vi "Check_Execution_Row.vi"(0 "Execution Row":T1 {"Row Duration (mins)" format="%#.1f"; "Row No" min=0; "Trace Gas Concentration (%)" min=0.0 format="%#.2f"; "Emission Rate (l/min)" format="%#.2f"; "Tunnel Speed" format="%#.2f"; "Start X" format="%#.2f"; "Start Y" format="%#.2f"; "Start Z" format="%#.2f"; "End X" format="%#.2f"; "End Y" format="%#.2f"; "End Z" format="%#.2f"; "Averaging time (min)" min=0.0 format="%#.2f"}, 3 "Synchronization Start No":i32=1 min=1 max=100, 4 "Row Index":i32, 5 "Max Tunnel Speed":dbl format="%.2f") -> (6 "Editted Row":bool, 7 "Execution Row Out":T1 {"Row Duration (mins)" format="%#.1f"; "Row No" min=0; "Trace Gas Concentration (%)" min=0.0 format="%#.2f"; "Emission Rate (l/min)" format="%#.2f"; "Tunnel Speed" format="%#.2f"; "Start X" format="%#.2f"; "Start Y" format="%#.2f"; "Start Z" format="%#.2f"; "End X" format="%#.2f"; "End Y" format="%#.2f"; "End Z" format="%#.2f"; "Averaging time (min)" min=0.0 format="%#.2f"}, 9 "Continue?":bool, 10 "Error Comments":string)   [LabVIEW 2014]
uses:
  Traverse_cluster.ctl
  Spacing.ctl
  Controls/Multi_run_mode.ctl
  Controls/User_Specific_mode.ctl
  Controls/Home.ctl
  Controls/Tunnel_Coordinates.ctl
  ADAM Client/Sub VIs/ADAM Controls/Channel_names.ctl
  Globals/Extra_Commands_Global.vi
  Globals/Constants_global.vi
  Globals/Trav_pos_global.vi
panel:
  out "Traverse line Out":T1 {"Row Duration (mins)" format="%#.1f"; "Row No" min=0; "Trace Gas Concentration (%)" min=0.0 format="%#.2f"; "Emission Rate (l/min)" format="%#.2f"; "Tunnel Speed" format="%#.2f"; "Start X" format="%#.2f"; "Start Y" format="%#.2f"; "Start Z" format="%#.2f"; "End X" format="%#.2f"; "End Y" format="%#.2f"; "End Z" format="%#.2f"; "Averaging time (min)" min=0.0 format="%#.2f"}
  out "Fixed Axis":bool[](array[boolean])
  out "Filenames":string[](array[string])
  out "Current Sync Number":i32
  out "Checks":string[](array[string])
  in  "Edit in Excel":bool
  in  "OK":bool
  # "X           Y            Z"
  # "Start"
  # "End"
  # "X           Y            Z"
  # "Start"
  # "End"
  # "X           Y            Z"
  # "Start"
  # "End"
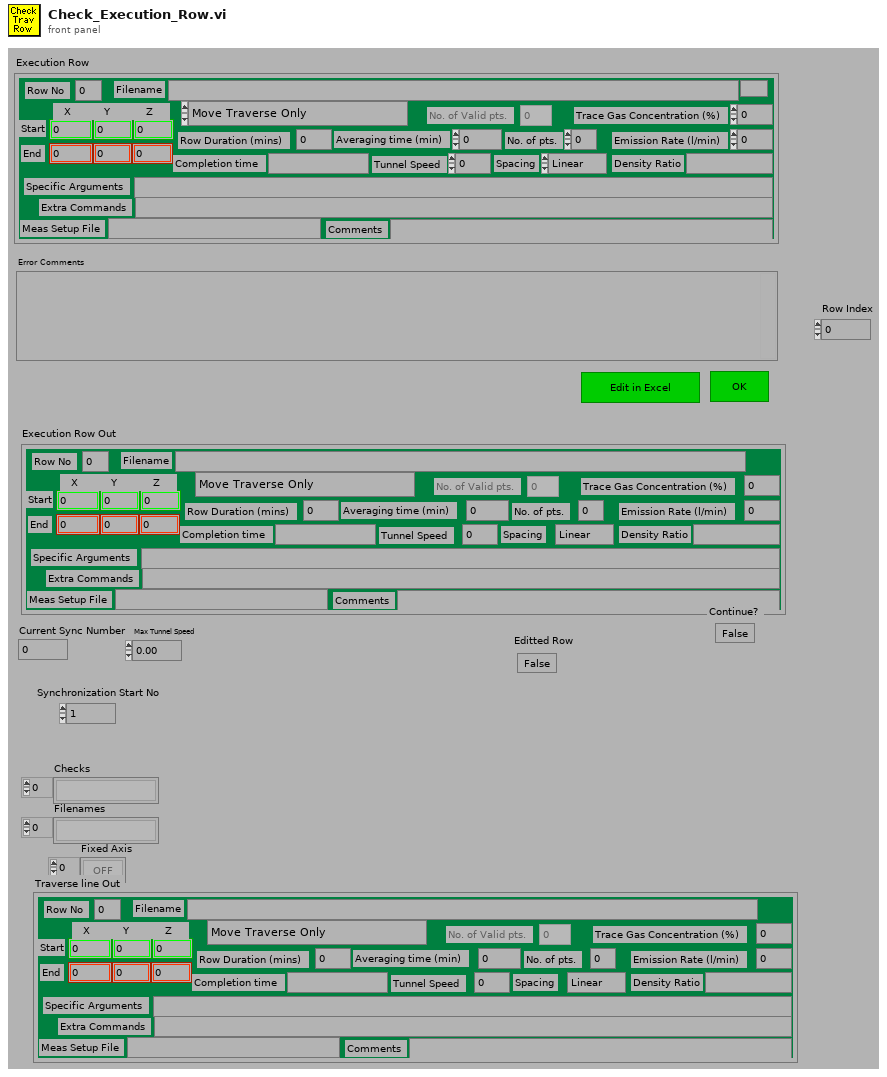
[diagram p1: front panel]
types:
  T1 = typedef "Traverse_cluster.ctl" = cluster{"Start X":dbl, "Start Y":dbl, "Start Z":dbl, "End X":dbl, "End Y":dbl, "End Z":dbl, "No. of pts.":i32, "Spacing":T2, "Filename":path, "Tunnel Speed":dbl, "Averaging time (min)":dbl, "Extra Commands":string, "Specific Arguments":string, "Emission Rate (l/min)":dbl, "Trace Gas Concentration (%)":dbl, "Density Ratio":string, "Comments":string, "Row No":i32, "Row Type Selector":T3, "Completion time":string, "Row Duration (mins)":dbl, "No. of Valid pts.":i32, "Meas Setup File":string}
  T2 = typedef "Spacing.ctl" = enum16{"Linear", "Log", "Gauss", "Specified", "N/A"}
  T3 = typedef "Multi_run_mode.ctl" = enum16{"Move Traverse Only", "Set Tunnel Speed Only", "Set Source Only", "Set Measurement Conditions", "Single Measurement", "Vertical Profile", "Lateral Profile", "Longitudinal Profile", "Explore Volume", "Multi-Axis Profile", "Auto Calibrate", "Meas Fast FID Bkgnd", "Check Beam Power", "Scanning Valve Measurement", "Run VI Named:", "Set ADAM Ch", "Wait (minutes)", "Send Message", "Synchronize With:", "Fall Back to this Row", "Turn Off Row Repeating", "Blank Row", "Traverse 3D Volume"}
  T4 = enum16{"All Channel Names", "Valid Channel Names"}
  T5 = typedef "User_Specific_mode.ctl" = enum16{"Check VI only", "Run VI"}
  T6 = typedef "Home.ctl" = enum16{"Don't Home", "Home  +X", "Home  -X", "Home  +Y", "Home  -Y", "Home  +Z", "Home  -Z"}
  T7 = typedef "Tunnel_Coordinates.ctl" = enum16{"Work in Tunnel Coordinates", "Work in Model Coordinates"}
  T8 = enum16{"Zero or one", "One", "Zero or more", "One or more"}
  T9 = typedef "Channel_names.ctl" = enum16{"Active Only", "Active + Off", "All Channels"}
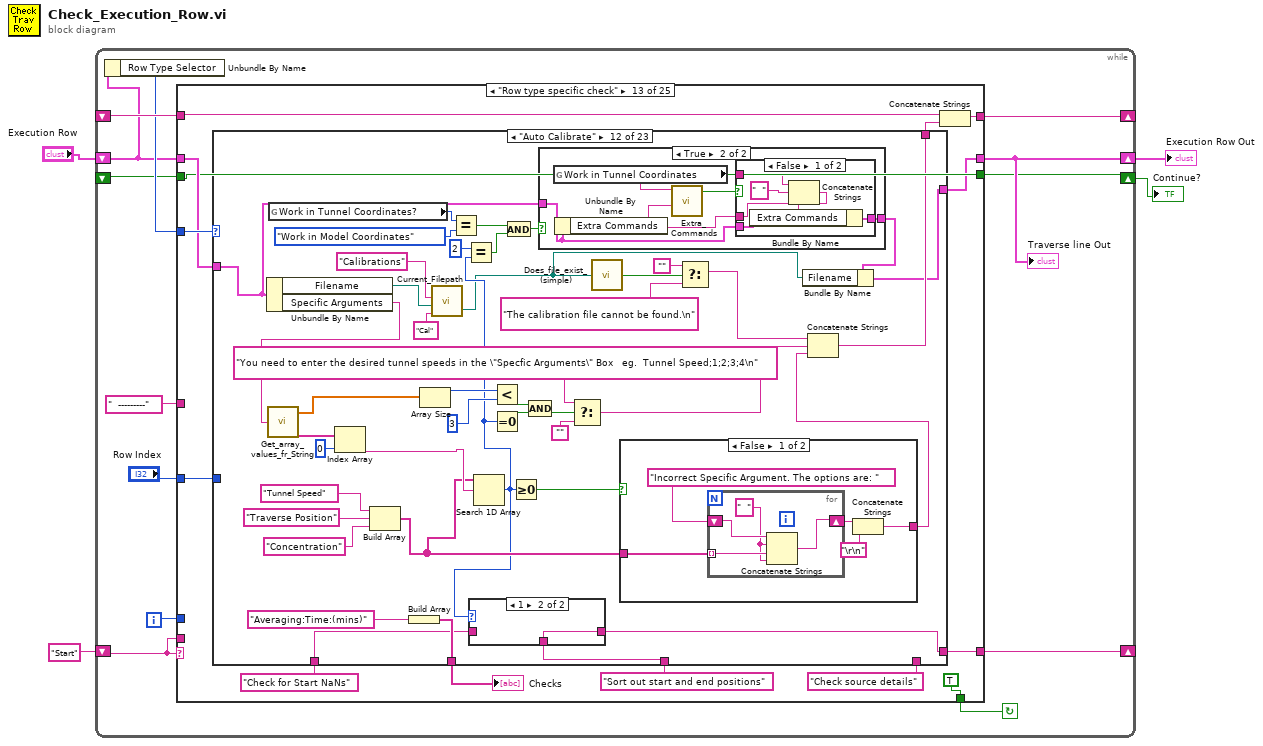
[diagram p0: block diagram]
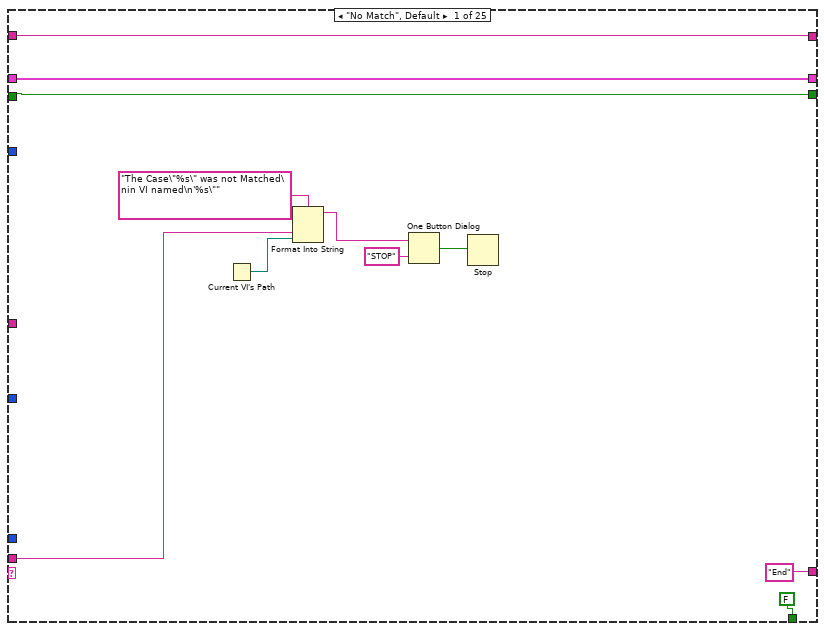
[diagram p2: hidden frame]
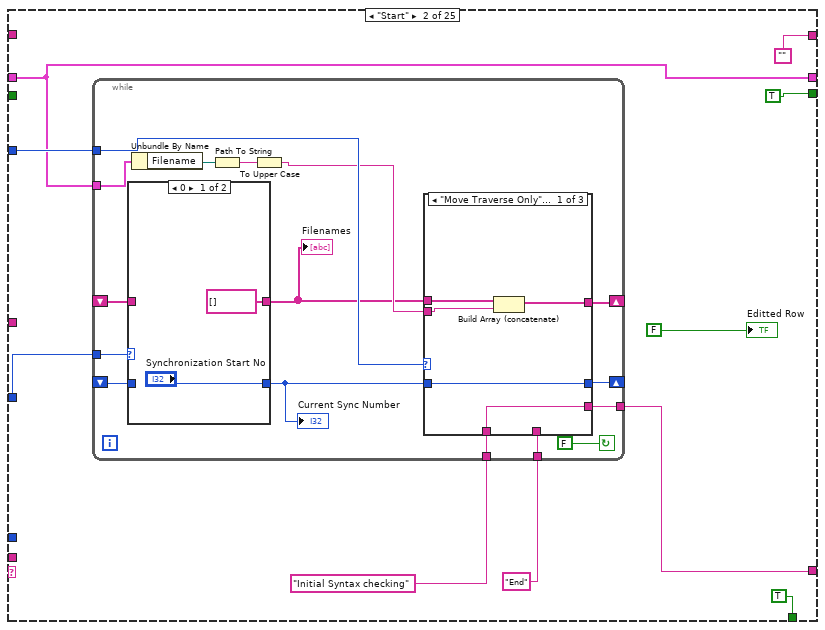
[diagram p3: hidden frame]
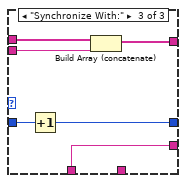
[diagram p6: hidden frame]
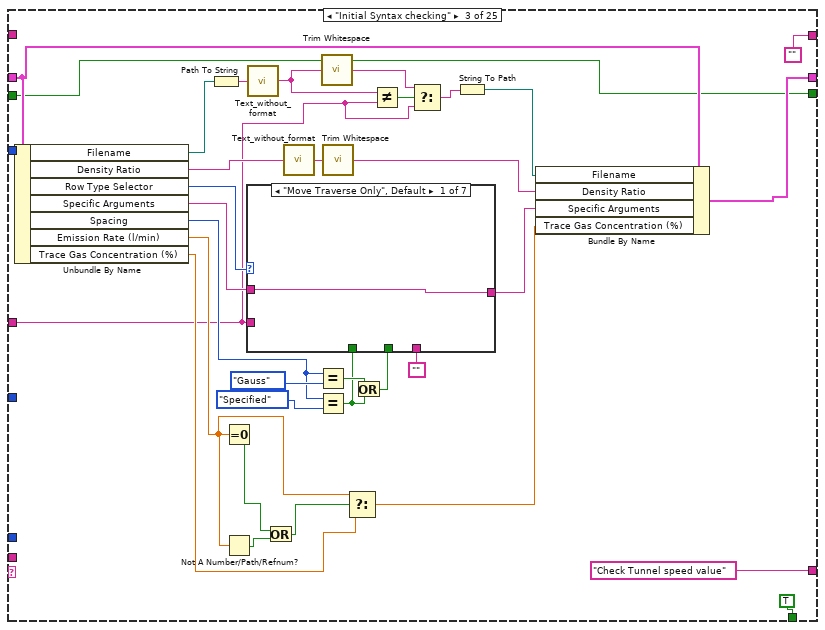
[diagram p7: hidden frame]
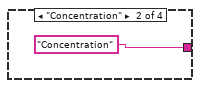
[diagram p9: hidden frame]
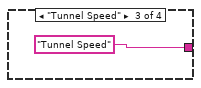
[diagram p10: hidden frame]
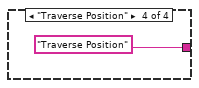
[diagram p11: hidden frame]
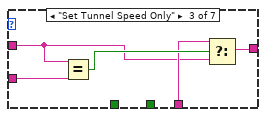
[diagram p12: hidden frame]
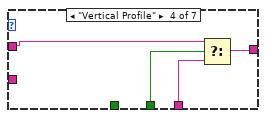
[diagram p13: hidden frame]
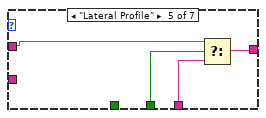
[diagram p14: hidden frame]
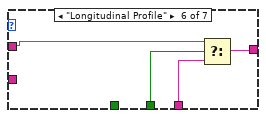
[diagram p15: hidden frame]
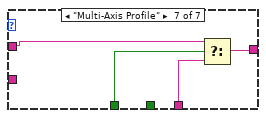
[diagram p16: hidden frame]
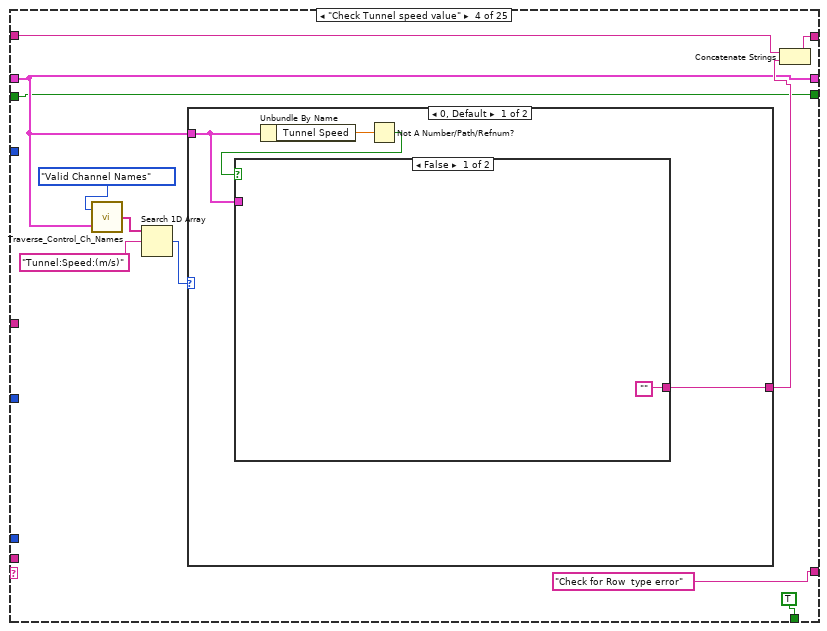
[diagram p17: hidden frame]
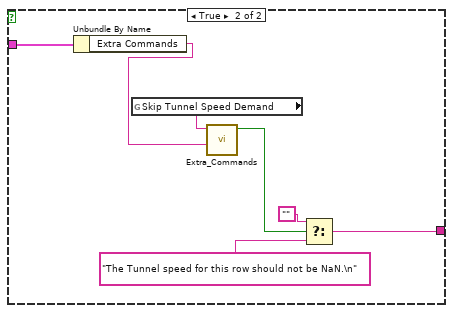
[diagram p18: hidden frame]
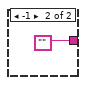
[diagram p19: hidden frame]
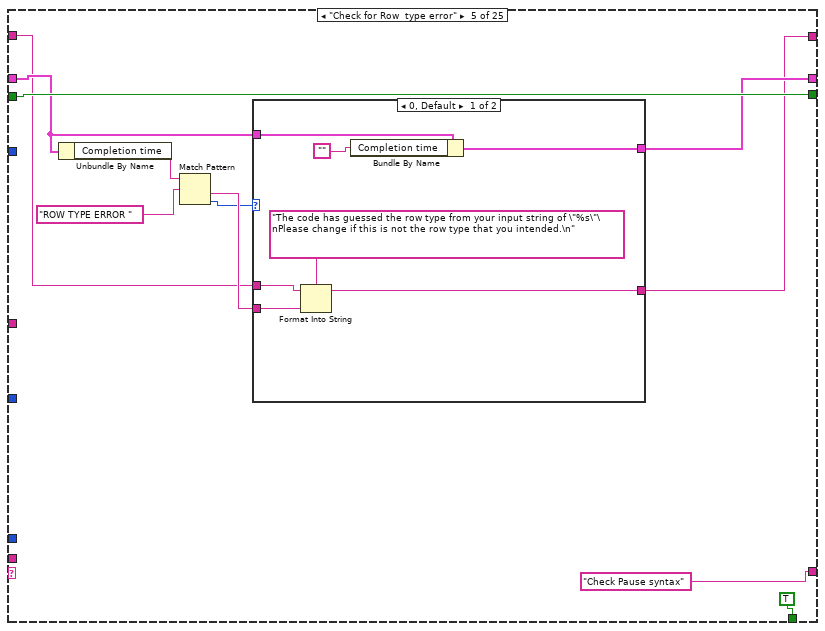
[diagram p20: hidden frame]
diagram:
  n1 = while {
    shift-left: _ -> [w16]
    shift-right: [w17] -> _
    shift-left: "Start" -> [w9]
    shift-right: [w14] -> _
    shift-right: [w8] -> w2
    shift-left: "Execution Row" -> [w5]
    shift-right: [w7] -> w1
    shift-left: _ -> [w6]
    i -> [w10]
    stop <- w15 continue-if-true
    n2 = Unbundle By Name(w5) -> ("Row Type Selector"=w12:T3)
    n3 = case shown="\"Row type specific check\"" w9 {
      tunnel: w5 -> [w22 w32 w100 w137 w161 w193 w218 w269 w316 w372 w405 w413 w452 w811 w911 w948 w976 w1061 w1093 w1103 w1173 _ w1212 w1219 w1229]
      tunnel: "  ---------" ("f") -> [_ _ w74 _ _ w197 _ _ _ _ _ _ _ _ _ _ _ _ _ _ _ _ _ _ _]
      tunnel: "Row Index" -> [_ w36 _ _ _ _ w215 _ _ _ _ _ w446 _ _ _ _ _ _ _ _ _ w1213 _ w1228]
      tunnel: [w21 "" "" w138 w158 w186 w224 w274 w321 w374 w409 w418 w456 w816 w921 w954 w999 w1059 w1097 w1104 w1179 w1190 w1214 w1224 w1231] -> w17
      tunnel: w12 -> [_ w35 _ _ _ w179 _ _ _ _ _ w416 w455 w812 w909 _ _ _ _ w1108 _ _ _ _ _]
      tunnel: w16 -> [w21 _ _ w139 w159 w188 w225 w275 w322 w374 w408 w419 w457 w816 w922 w955 w1000 w1059 w1098 w1109 w1179 w1190 w1214 w1224 w1231]
      tunnel: [FALSE TRUE TRUE TRUE TRUE TRUE TRUE TRUE TRUE TRUE TRUE TRUE TRUE TRUE TRUE TRUE TRUE TRUE TRUE w1100 TRUE TRUE TRUE TRUE FALSE] -> w15
      tunnel: ["End" w33 "Check Tunnel speed value" ("f") "Check for Row  type error" ("f") "Check Pause syntax" ("f") w191 "Check Traverse Setup Name" ("f") "Check IF command" ("f") "Check Measurement Setup?" ("f") w376 "Check Maximum tunnel speed" ("f") "Row type specific check" ("f") w453 "Check for position NaNs" ("f") w912 "Check source details" ("t") "Check source details" ("f") w1056 "check entered filename etc" ("f") w1106 "What to do next?" ("f") w1188 "Initial Syntax checking" "End" "End"] -> w14
      tunnel: w10 -> [_ _ _ _ _ _ _ _ _ _ _ _ _ _ _ _ _ _ _ _ _ _ _ _ _]
      tunnel: w9 -> [w23 _ _ _ _ _ _ _ _ _ _ _ _ _ _ _ _ _ _ _ _ _ _ _ _]
      tunnel: [w22 w32 w77 w137 w162 w181 w217 w269 w316 w372 w404 w413 w447 w810 w911 w948 w975 w1060 w1093 w1102 w1173 w1181 w1215 w1219 w1227] -> w8
      tunnel: [w18 TRUE w75 w136 w168 w182 w219 w267 w313 w378 w406 w411 w449 w808 w910 w947 w973 w1064 w1091 w1100 w1172 w1180 w1209 w1218 w1225] -> w7
      tunnel: w6 -> [w18 _ w75 w136 w168 w182 w219 w267 w313 w378 w406 w411 w449 w808 w910 w947 w973 w1064 w1091 _ w1172 _ w1209 w1218 w1225]
      frame "No Match", Default {
        n4 = Current VI's Path() -> (path=w24:path)
        n5 = Format Into String(format string="The Case\"%s\" was not Matched\nin VI named\n'%s\"" ("Format String"), w23, w24) -> (resulting string=w27:string)  [unwired: 2 in, 1 out]
        n6 = One Button Dialog(message=w27, button name ("OK")="STOP") -> (true=w25:bool)
        n7 = Stop(stop? (T)=w25) -> ()
      }
      frame "Start" {
        n8 = while {
          tunnel: "End" -> [w40]
          tunnel: "Initial Syntax checking" -> [w41]
          tunnel: [w42] -> w33
          tunnel: w32 -> [w49]
          shift-left: _ -> [w48]
          shift-right: [w47] -> _
          tunnel: w35 -> [w53]
          shift-left: _ -> [w52]
          shift-right: [w51] -> _
          tunnel: w36 -> [w54]
          stop <- FALSE continue-if-true
          n9 = case shown="0" w54 {
            tunnel: ["Synchronization Start No" w58] -> w50
            tunnel: w52 -> [_ w58]
            tunnel: w48 -> [_ w57]
            tunnel: [string[] [] w57] -> w43
            frame 0 {
            }
            frame 1, Default {
            }
          }
          "Current Sync Number" <- w50
          "Filenames" <- w43
          n10 = Unbundle By Name(w49) -> ("Filename"=w46:path)
          n11 = Path To String(path=w46) -> (string=w45:string)
          n12 = To Upper Case(1:w45) -> (0:w44:string)
          n13 = case shown="\"Move Traverse Only\", Default" w53 {
            tunnel: w50 -> [w63 w66 w72]
            tunnel: [w63 w66 w71] -> w51
            tunnel: w44 -> [w61 _ w70]
            tunnel: w43 -> [w62 w65 w69]
            tunnel: [w60 w65 w68] -> w47
            tunnel: [w59 w64 w67] -> w42
            tunnel: w41 -> [w59 _ w67]
            tunnel: w40 -> [_ w64 _]
            frame "Move Traverse Only", Default {
              n14 = Build Array (concatenate)(w62, w61) -> (w60:string[])
            }
            frame "Blank Row" {
            }
            frame "Synchronize With:" {
              n15 = Increment(x=w72) -> (x+1=w71:i32)
              n16 = Build Array (concatenate)(w69, w70) -> (w68:string[])
            }
          }
        }
        "Editted Row" <- FALSE ("Editted Row")
      }
      frame "Initial Syntax checking" {
        n17 = Unbundle By Name(w100) -> ("Filename"=w73:path, "Density Ratio"=w79:string, "Row Type Selector"=w97:T3, "Specific Arguments"=w95:string, "Spacing"=w87:T2, "Emission Rate (l/min)"=w83:dbl, "Trace Gas Concentration (%)"=w93:dbl)
        n18 = Path To String(path=w73) -> (string=w81:string)
        n19 = Equal To 0?(x=w83) -> (x = 0?=w85:bool)
        n20 = Not A Number/Path/Refnum?(number/path/refnum=w83) -> (NaN/Path/Refnum?=w84:bool)
        n21 = call "Text_without_format.vi"("Input string"=w81) -> ("Output string"=w104:string)
        n22 = Or(x=w85, y=w84) -> (x .or. y?=w82:bool)
        n23 = call "Text_without_format.vi"("Input string"=w79) -> ("Output string"=w99:string)
        n24 = Equal?(x=w87, y=Spacing."Gauss" ("Spacing")) -> (x = y?=w89:bool)
        n25 = Equal?(x=w87, y=Spacing."Specified" ("Spacing")) -> (x = y?=w86:bool)
        n26 = call <vilib>:"Trim Whitespace.vi"("string"=w104) -> ("trimmed string"=w103:string)  [unwired: 1 in]
        n27 = call <vilib>:"Trim Whitespace.vi"("string"=w99) -> ("trimmed string"=w78:string)  [unwired: 1 in]
        n28 = Select(t=w83, s=w82, f=w93) -> (s? t:f=w92:dbl)
        n29 = Or(x=w89, y=w86) -> (x .or. y?=w88:bool)
        n30 = case shown="\"Move Traverse Only\", Default" w97 {
          tunnel: [w106 w108 w113 w119 w123 w127 w131] -> w96
          tunnel: w95 -> [w106 w107 w114 w121 w125 w129 w133]
          tunnel: "" -> [_ _ w115 w120 w124 w128 w132]
          tunnel: w88 -> [_ _ _ w118 w122 w126 _]
          tunnel: w86 -> [_ _ _ _ _ _ w130]
          tunnel: w74 -> [_ _ w117 _ _ _ _]
          frame "Move Traverse Only", Default {
          }
          frame "Auto Calibrate" {
            n31 = case shown="\"No Match\", Default" w107 {
              tunnel: [w109 "Concentration" "Tunnel Speed" "Traverse Position"] -> w108
              tunnel: w107 -> [w109 _ _ _]
              frame "No Match", Default {
              }
              frame "Concentration" {
              }
              frame "Tunnel Speed" {
              }
              frame "Traverse Position" {
              }
            }
          }
          frame "Set Tunnel Speed Only" {
            n32 = Equal?(x=w114, y=w117) -> (x = y?=w116:bool)
            n33 = Select(t=w115, s=w116, f=w114) -> (s? t:f=w113:string)
          }
          frame "Vertical Profile" {
            n34 = Select(t=w121, s=w118, f=w120) -> (s? t:f=w119:string)
          }
          frame "Lateral Profile" {
            n35 = Select(t=w125, s=w122, f=w124) -> (s? t:f=w123:string)
          }
          frame "Longitudinal Profile" {
            n36 = Select(t=w129, s=w126, f=w128) -> (s? t:f=w127:string)
          }
          frame "Multi-Axis Profile" {
            n37 = Select(t=w133, s=w130, f=w132) -> (s? t:f=w131:string)
          }
        }
        n38 = Not Equal?(x=w104, y=w74) -> (x != y?=w105:bool)
        n39 = Select(t=w103, s=w105, f=w74) -> (s? t:f=w102:string)
        n40 = String To Path(string=w102) -> (path=w80:path)
        n41 = Bundle By Name(cluster=w100, "Filename"=w80, "Density Ratio"=w78, "Specific Arguments"=w96, "Trace Gas Concentration (%)"=w92) -> (w77:T1)
      }
      frame "Check Tunnel speed value" {
        n42 = call "Traverse_Control_Ch_Names.vi"("Traverse line"=w137, "Mode"=T4."Valid Channel Names") -> ("Channel names"=w143:string[])
        n43 = Search 1D Array(1D array=w143, element="Tunnel:Speed:(m/s)" ("Label for value")) -> (index of element=w141:i32)  [unwired: 1 out]
        n44 = case shown="0, Default" w141 {
          tunnel: w137 -> [w146 _]
          tunnel: [w145 ""] -> w140
          frame 0, Default {
            n45 = Unbundle By Name(w146) -> ("Tunnel Speed"=w148:dbl)
            n46 = Not A Number/Path/Refnum?(number/path/refnum=w148) -> (NaN/Path/Refnum?=w147:bool)
            n47 = case shown="False" w147 {
              tunnel: w146 -> [_ w156]
              tunnel: ["" w150] -> w145
              frame False {
              }
              frame True {
                n48 = Unbundle By Name(w156) -> ("Extra Commands"=w154:string)
                n49 = global read "Extra_Commands_Global.vi" "Skip Tunnel Speed Demand"() -> (w155:string)
                n50 = call "Extra_Commands.vi"("String to Search"=w154, "Command"=w155) -> ("Command Found"=w153:bool)  [unwired: 1 in, 4 out]
                n51 = Select(t="", s=w153, f="The Tunnel speed for this row should not be NaN.\n") -> (s? t:f=w150:string)
              }
            }
          }
          frame -1 {
          }
        }
        n52 = Concatenate Strings(w139, w140) -> (w138:string)
      }
      frame "Check for Row  type error" {
        n53 = Unbundle By Name(w161) -> ("Completion time"=w164:string)
        n54 = Match Pattern(string=w164, regular expression="ROW TYPE ERROR " ("format string")) -> (after substring=w163:string, offset past match=w160:i32)  [unwired: 3 out]
        n55 = case shown="0, Default" w160 {
          tunnel: w163 -> [w175 _]
          tunnel: [w173 w177] -> w162
          tunnel: w161 -> [w172 w177]
          tunnel: [w170 w176] -> w158
          tunnel: w159 -> [w169 w176]
          frame 0, Default {
            n56 = Format Into String(format string="The code has guessed the row type from your input string of \"%s\"\nPlease change if this is not the row type that you intended.\n", initial string=w169, w175) -> (resulting string=w170:string)  [unwired: 1 in, 1 out]
            n57 = Bundle By Name(cluster=w172, "Completion time"="") -> (w173:T1)
          }
          frame -1 {
          }
        }
      }
      frame "Check Pause syntax" {
        n58 = Unbundle By Name(w193) -> ("Extra Commands"=w198:string)
        n59 = Equal?(x=Multi_run_mode."Set ADAM Ch" ("Row Type Selector"), y=w179) -> (x = y?=w178:bool)
        n60 = Not Equal?(x=w198, y=w197) -> (x != y?=w199:bool)
        n61 = Select(t=w198, s=w199, f="") -> (s? t:f=w195:string)
        n62 = call <vilib>:"Trim Whitespace.vi"("string"=w195) -> ("trimmed string"=w190:string)  [unwired: 1 in]
        n63 = case shown="True" w178 {
          tunnel: [w201 TRUE] -> w192
          tunnel: w190 -> [w200 _]
          frame False {
            n64 = Equal?(x=w200, y="") -> (x = y?=w201:bool)
          }
          frame True {
          }
        }
        n65 = call "Pause_for_server_ch_val.vi"("Extra command string"=w190, "Simulate/Run"=User_Specific_mode."Check VI only") -> ("Extra command string Out"=w189:string, "Error Comments"=w187:string)
        n66 = Bundle By Name(cluster=w193, "Extra Commands"=w189) -> (w181:T1)
        n67 = Concatenate Strings(w188, w187) -> (w186:string)
        n68 = Select(t="Check Measurement Setup?", s=w192, f="Check Extra Commands") -> (s? t:f=w191:string)
      }
      frame "Check Extra Commands" {
        n69 = global read "Extra_Commands_Global.vi" "Home"() -> (w204:string)
        n70 = Unbundle By Name(w218) -> ("Extra Commands"=w210:string)
        n71 = for {
          N: 4 -> [_]
          tunnel: w210 -> [w243]
          shift-right: [w239] -> w205
          shift-left: "" -> [w240]
          i -> [w245]
          n72 = case shown="3" w245 {
            tunnel: [w248 w250 w252 w254] -> w242
            tunnel: ["The Extra Command \"%s\" should have a numeric argument of (Centre; Intensity) eg 0 ; 0.85 for Gaussian spacing or (Offset) eg 300 for Log \n" ("Format String") "The Extra Command \"%s\" should have a numeric argument.\n" ("Format String") "The Extra Command \"%s\" should have a numeric argument.\n" ("Format String") "The Extra Command \"%s\" should have a numeric argument greater than Zero.\n" ("Format String")] -> w237
            frame 0, Default {
              n73 = global read "Extra_Commands_Global.vi" "Point Spacing Parameters"() -> (w248:string)
            }
            frame 1 {
              n74 = global read "Extra_Commands_Global.vi" "Establish Exp Conditions (s)"() -> (w250:string)
            }
            frame 2 {
              n75 = global read "Extra_Commands_Global.vi" "Minutes Before Repeating Row"() -> (w252:string)
            }
            frame 3 {
              n76 = global read "Extra_Commands_Global.vi" "Puff Duration Sec"() -> (w254:string)
            }
          }
          n77 = call "Extra_Commands.vi"("String to Search"=w243, "Command"=w242) -> ("String Value"=w244:string, "Command Found"=w246:bool)  [unwired: 1 in, 3 out]
          n78 = case shown="True" w246 {
            tunnel: w244 -> [_ w263]
            tunnel: w242 -> [_ w261]
            tunnel: [w255 w258] -> w241
            tunnel: "" -> [w255 w257]
            tunnel: w237 -> [_ w256]
            frame False {
            }
            frame True {
              n79 = Decimal String To Number(string=w263) -> (offset past number=w262:i32)  [unwired: 3 out]
              n80 = Equal To 0?(x=w262) -> (x = 0?=w260:bool)
              n81 = Format Into String(format string=w256, w261) -> (resulting string=w259:string)  [unwired: 2 in, 1 out]
              n82 = Select(t=w259, s=w260, f=w257) -> (s? t:f=w258:string)
            }
          }
          n83 = Concatenate Strings(w241, w240) -> (w239:string)
        }
        n84 = call "Extra_Commands.vi"("String to Search"=w210, "Command"=w204) -> ("String Value"=w208:string, "Command Found"=w209:bool)  [unwired: 1 in, 3 out]
        n85 = case shown="True" w209 {
          tunnel: w208 -> [_ w236]
          tunnel: [TRUE w233] -> w207
          frame False {
          }
          frame True {
            n86 = call "Home_String_to_Enumerated_Type.vi"("String"=w236) -> ("Home"=w235:T6)
            n87 = Not Equal?(x=w235, y=Home."Don't Home" ("Home")) -> (x != y?=w233:bool)
          }
        }
        n88 = call "Trav_Prog_Extra_Commands.vi"() -> ("Extra Commands Array"=w220:string[])  [unwired: 2 out]
        n89 = call "Valid_Extra_Command.vi"("Extra Commands string"=w210, "Valid Commands Array"=w220) -> ("Output String"=w223:string, "Extra Commands string Out"=w216:string)  [unwired: 3 out]
        n90 = Bundle By Name(cluster=w218, "Extra Commands"=w216) -> (w217:T1)
        n91 = call "Skip_If Sd_Error_Below.vi"("String to Search"=w216, "Simulate/Run"=User_Specific_mode."Check VI only", "Measurement setup Applied?"=FALSE, "Row Number"=w215) -> ("Error String"=w212:string)  [unwired: 1 in, 4 out]
        n92 = case shown="False" w207 {
          tunnel: [w229 w231] -> w206
          tunnel: w205 -> [w228 w231]
          tunnel: w204 -> [w230 _]
          frame False {
            n93 = Format Into String(format string="The Extra Command \"%s\" argument should be either\nHome  +X\nHome  -X\nHome  +Y\nHome  -Y\nHome  +Z\nHome  -Z\n" ("Format String"), initial string=w228, w230) -> (resulting string=w229:string)  [unwired: 1 in, 1 out]
          }
          frame True {
          }
        }
        n94 = Concatenate Strings(w225, w223, w206, w212) -> (w224:string)
      }
      frame "Check Traverse Setup Name" {
        n95 = Unbundle By Name(w269) -> ("Extra Commands"=w266:string)
        n96 = global read "Extra_Commands_Global.vi" "!Traverse Setup"() -> (w272:string)
        n97 = call "Extra_Commands.vi"("String to Search"=w266, "Command"=w272) -> ("String Value"=w270:string, "Command Found"=w271:bool)  [unwired: 1 in, 3 out]
        n98 = case shown="True" w271 {
          tunnel: w270 -> [_ w286]
          tunnel: [w276 w282] -> w268
          tunnel: "" -> [w276 w281]
          frame False {
          }
          frame True {
            n99 = call "Get_array_values_fr_String.vi"("String Value"=w286) -> ("String array"=w278:string[])  [unwired: 1 out]
            n100 = global read "Constants_global.vi" "Traverse folder"() -> (w287:path)
            n101 = Empty Array?(array=w278) -> (empty?=w279:bool)
            n102 = Select(t=string[] [""], s=w279, f=w278) -> (s? t:f=w280:string[])
            n103 = List Folder(path=w287) -> (folder names=w284:string[])  [unwired: 1 in, 5 out]
            n104 = for {
              tunnel: w280 -> [w303] mode=indexing
              tunnel: w284 -> [w305]
              shift-right: [w301] -> w285
              shift-left: w281 -> [w302]
              n105 = Search 1D Array(1D array=w305, element=w303) -> (index of element=w304:i32)  [unwired: 1 out]
              n106 = case shown="-1" w304 {
                tunnel: w303 -> [_ w309]
                tunnel: [w306 w308] -> w301
                tunnel: w302 -> [w306 w307]
                frame Default {
                }
                frame -1 {
                  n107 = Format Into String(format string="%s is not a valid Travese setup.\n", initial string=w307, w309) -> (resulting string=w308:string)  [unwired: 1 in, 1 out]
                }
              }
            }
            n108 = Empty String/Path?(string/path=w285) -> (empty?=w283:bool)
            n109 = case shown="False" w283 {
              tunnel: w284 -> [w294 _]
              tunnel: [w293 w300] -> w282
              tunnel: w285 -> [w291 w300]
              frame False {
                w288 = "\r\n"
                n110 = Concatenate Strings(w291, " Valid option are:" ("format string"), w288) -> (w290:string)
                n111 = for {
                  shift-right: [w297] -> w293
                  shift-left: w290 -> [w298]
                  tunnel: w294 -> [w299] mode=indexing
                  tunnel: "!Traverse Setup =  " ("Substring") -> [w296]
                  tunnel: w288 -> [w295]
                  n112 = Concatenate Strings(w298, w296, w299, w295) -> (w297:string)
                }
              }
              frame True {
              }
            }
          }
        }
        n113 = Concatenate Strings(w275, w268) -> (w274:string)
      }
      frame "Check IF command" {
        n114 = Unbundle By Name(w316) -> ("Extra Commands"=w312:string)
        n115 = global read "Extra_Commands_Global.vi" "If Command"() -> (w319:string)
        n116 = call "Extra_Commands.vi"("String to Search"=w312, "Command"=w319) -> ("String Value"=w317:string, "Command Found"=w318:bool)  [unwired: 1 in, 3 out]
        n117 = case shown="False" w318 {
          tunnel: w317 -> [_ w328]
          tunnel: [w323 w327] -> w314
          tunnel: "" -> [w323 w325]
          frame False {
          }
          frame True {
            n118 = call "Get_array_values_fr_String.vi"("String Value"=w328) -> ("Numeric Array"=w324:dbl[], "String array"=w326:string[])
            n119 = Index Array(array=w326, index=0 ("Index")) -> (element=w329:string)
            n120 = case shown="\"Global Value Between\"" w329 {
              tunnel: w328 -> [w334 _ _ _]
              tunnel: [w333 w359 w360 "The !If  command has not been recognised.\nExtra command Example:\n!IF = Time Between;10:45;and;14:00;Execute Row (or) Skip Row\n\n!IF = ADAM Channel Between;Channel Name; 0.5;1.0\n\n!IF = Global Value Between; 0.5;1.0" ("Error Comments")] -> w327
              tunnel: w326 -> [_ w350 w368 _]
              tunnel: w325 -> [_ w343 w361 _]
              tunnel: w324 -> [_ _ _ _]
              frame "Time Between" {
                n121 = Get Date/Time In Seconds() -> (seconds since 1Jan1904=w331:timestamp)
                n122 = To Double Precision Float(number=w331) -> (double precision float=w332:dbl)
                n123 = call "If_Time_arguments.vi"("seconds since 1Jan1904"=w332, "String Value"=w334) -> ("Error Comments"=w333:string)  [unwired: 2 out]
              }
              frame "ADAM Channel Between" {
                n124 = Index Array(array=w350, index=1 ("Index")) -> (element=w353:string)
                n125 = Index Array(array=w350, index=2 ("Index")) -> (element=w349:string)
                n126 = Index Array(array=w350, index=3 ("Index")) -> (element=w348:string)
                n127 = Build Array(w353) -> (w355:string[])
                n128 = Decimal Digit?(1:w349) -> (0:w346:bool)
                n129 = Decimal Digit?(1:w348) -> (0:w347:bool)
                n130 = call "Get_Current_Scan_client.vi"("ADAM Ch Names"=w355) -> ("Numerical Values"=w357:dbl[])  [unwired: 3 out]
                n131 = And(x=w346, y=w347) -> (x .and. y?=w345:bool)
                n132 = Index Array(array=w357, index=0 ("Index")) -> (element=w358:dbl)
                n133 = Select(t=w343, s=w345, f="you must give two limits\n") -> (s? t:f=w339:string)
                n134 = Not A Number/Path/Refnum?(number/path/refnum=w358) -> (NaN/Path/Refnum?=w342:bool)
                n135 = Select(t="Invalid ADAM Channel Name\n", s=w342, f=w343) -> (s? t:f=w340:string)
                n136 = Concatenate Strings(w340, w339) -> (w337:string)
                n137 = Concatenate Strings(w337, "Extra command Example:\n!IF = ADAM Channel Between;Channel Name; 0.5;1.0") -> (w336:string)
                n138 = Empty String/Path?(string/path=w337) -> (empty?=w338:bool)
                n139 = Select(t=w343, s=w338, f=w336) -> (s? t:f=w359:string)
              }
              frame "Global Value Between" {
                n140 = Index Array(array=w368, index=1 ("Index")) -> (element=w367:string)
                n141 = Index Array(array=w368, index=2 ("Index")) -> (element=w366:string)
                n142 = Decimal Digit?(1:w367) -> (0:w364:bool)
                n143 = Decimal Digit?(1:w366) -> (0:w365:bool)
                n144 = And(x=w364, y=w365) -> (x .and. y?=w363:bool)
                n145 = Select(t=w361, s=w363, f="The Extra command IF statement must have two numerical values for the limits\n\nExtra command Example:\n!IF = Global Value Between; 0.5;1.0") -> (s? t:f=w360:string)
              }
              frame "No Match", Default {
              }
            }
          }
        }
        n146 = Concatenate Strings(w322, w314) -> (w321:string)
      }
      frame "Check Measurement Setup?" {
        n147 = Unbundle By Name(w372) -> ("Row Type Selector"=w377:T3, "Specific Arguments"=w375:string)
        n148 = case shown="\"Traverse 3D Volume\"" w377 {
          tunnel: ["Check Measurement Setup" ("t") "Check Measurement Setup" ("t") "Check Measurement Setup" ("t") "Check Measurement Setup" ("t") "Check Measurement Setup" ("t") "Check Measurement Setup" ("t") "Check Measurement Setup" ("t") "Check Measurement Setup" ("t") "Check Measurement Setup" ("t") "Check Measurement Setup" ("t") "Check Measurement Setup" ("t") w391 w400] -> w376
          tunnel: w375 -> [_ _ _ _ _ _ _ _ _ _ _ w398 _]
          tunnel: "Check Maximum tunnel speed" ("f") -> [_ _ _ _ _ _ _ _ _ _ _ w392 w400]
          tunnel: w372 -> [_ _ _ _ _ _ _ _ _ _ _ w395 _]
          frame "Lateral Profile" {
          }
          frame "Traverse 3D Volume" {
          }
          frame "Longitudinal Profile" {
          }
          frame "Explore Volume" {
          }
          frame "Multi-Axis Profile" {
          }
          frame "Vertical Profile" {
          }
          frame "Single Measurement" {
          }
          frame "Scanning Valve Measurement" {
          }
          frame "Auto Calibrate" {
          }
          frame "Meas Fast FID Bkgnd" {
          }
          frame "Check Beam Power" {
          }
          frame "Run VI Named:" {
            n149 = Match Pattern(string=w398, regular expression=";") -> (before substring=w397:string)  [unwired: 4 out]
            n150 = call <vilib>:"Trim Whitespace.vi"("string"=w397) -> ("trimmed string"=w396:string)  [unwired: 1 in]
            n151 = call "Run_VI_Named_specific.vi"("Run VI Named String"=w396, "Multi Run Row"=w395) -> ("Check Meas Setup?"=w394:bool)  [unwired: 9 out]
            n152 = Select(t="Check Measurement Setup", s=w394, f=w392) -> (s? t:f=w391:string)
          }
          frame "Set Tunnel Speed Only", Default {
          }
        }
      }
      frame "Check Measurement Setup" {
        n153 = Unbundle By Name(w405) -> ("Meas Setup File"=w403:string)
        n154 = call "Check_Measurement_Setups.vi"("Measurement Setup String"=w403) -> ("Measurement Setup String Out"=w402:string, "Error Comments"=w401:string)
        n155 = Bundle By Name(cluster=w405, "Meas Setup File"=w402) -> (w404:T1)
        n156 = Concatenate Strings(w408, w401) -> (w409:string)
      }
      frame "Check Maximum tunnel speed" {
        n157 = case shown="\"Set Tunnel Speed Only\", Default" w416 {
          tunnel: w413 -> [w438 _]
          tunnel: [w429 FALSE] -> w415
          tunnel: [w428 0.0] -> w414
          frame "Auto Calibrate" {
            n158 = Unbundle By Name(w438) -> ("Specific Arguments"=w437:string)
            n159 = call "Get_array_values_fr_String.vi"("String Value"=w437) -> ("Numeric Array"=w431:dbl[], "String array"=w436:string[])
            n160 = Index Array(array=w436, index=0 ("Index")) -> (element=w434:string)
            n161 = Equal?(x=w434, y="Tunnel Speed" ("Output Array")) -> (x = y?=w429:bool)
            n162 = Array Subset(array=w431, index=1 ("Array Index")) -> (w430:dbl[])  [unwired: 1 in]
            n163 = Array Max & Min(array=w430) -> (max value=w428:dbl)  [unwired: 3 out]
          }
          frame "Set Tunnel Speed Only", Default {
          }
        }
        n164 = case shown="False" w415 {
          tunnel: [w426 w427] -> w423
          tunnel: w413 -> [w425 _]
          tunnel: w414 -> [_ w427]
          frame False {
            n165 = Unbundle By Name(w425) -> ("Tunnel Speed"=w426:dbl)
          }
          frame True {
          }
        }
        n166 = Greater?(x=w423, y="Max Tunnel Speed") -> (0:w421:bool)
        n167 = Not A Number/Path/Refnum?(number/path/refnum=w423) -> (NaN/Path/Refnum?=w422:bool)
        n168 = Compound Arithmetic op=AND(invert w422, w421) -> (w420:bool)
        n169 = case shown="False" w420 {
          tunnel: w419 -> [w441 w443]
          tunnel: [w441 w442] -> w418
          tunnel: "Max Tunnel Speed" -> [_ w445]
          frame False {
          }
          frame True {
            n170 = Format Into String(format string="The maximum allowable tunnel speed is %.2f m/s.\n" ("Format String"), initial string=w443, w445) -> (resulting string=w442:string)  [unwired: 1 in, 1 out]
          }
        }
      }
      frame "Row type specific check" {
        n171 = case shown="\"Auto Calibrate\"" w455 {
          tunnel: w452 -> [w466 w475 w479 w483 w488 w493 w500 w507 w518 w526 w540 w545 w622 w629 w650 w687 w738 w766 w771 w775 w787 w791 w797]
          tunnel: [string[] [] string[] [] string[] [] string[] [] w489 w496 w503 w510 w523 w531 w541 w567 w624 string[] [] w667 string[] [] w733 string[] [] string[] [] string[] [] string[] [] string[] [] string[] []] -> w454
          tunnel: [w460 "" "" "" "" "" "" "" w519 w528 "" w581 w618 w628 w662 w683 w749 w768 "" w777 "" "" w799] -> w458
          tunnel: [w469 w476 w480 w484 w487 w494 w501 w508 w517 w527 w539 w566 w612 w627 w661 w690 w734 "check entered filename etc" "check entered filename etc" "check entered filename etc" "check entered filename etc" "check entered filename etc" "check entered filename etc"] -> w453
          tunnel: "Check source details" -> [_ w476 w480 _ _ _ _ _ _ _ w539 _ w612 w627 w661 w689 w735 _ _ _ _ _ _]
          tunnel: "Sort out start and end positions" -> [_ _ _ _ _ w494 w501 w508 _ w527 _ w564 _ _ _ _ _ _ _ _ _ _ _]
          tunnel: "Check for Start NaNs" -> [w469 _ _ w484 w487 _ _ _ w517 _ _ w565 _ _ _ _ _ _ _ _ _ _ _]
          tunnel: [w465 w475 w479 w483 w488 w493 w500 w507 w518 w526 w540 w546 w622 w637 w650 w686 w738 w766 w771 w775 w787 w791 w795] -> w447
          tunnel: w446 -> [_ _ _ _ _ _ _ _ _ _ _ _ _ _ _ w692 _ _ _ _ _ _ _]
          frame "Move Traverse Only" {
            n172 = Unbundle By Name(w466) -> ("Specific Arguments"=w467:string)
            n173 = call <vilib>:"Trim Whitespace.vi"("string"=w467) -> ("trimmed string"=w461:string)  [unwired: 1 in]
            n174 = Equal?(x=w461, y="No Backlash") -> (x = y?=w464:bool)
            n175 = Empty String/Path?(string/path=w461) -> (empty?=w463:bool)
            n176 = Or(x=w463, y=w464) -> (x .or. y?=w462:bool)
            n177 = case shown="True" w462 {
              tunnel: w461 -> [w472 _]
              tunnel: [w471 ""] -> w460
              frame False {
                n178 = Format Into String(format string="\"%s\" is an Incorrect Specific Argument. It should either be left blank or say \"No Backlash\"\n", w472) -> (resulting string=w471:string)  [unwired: 2 in, 1 out]
              }
              frame True {
              }
            }
            n179 = Bundle By Name(cluster=w466, "Specific Arguments"=w461) -> (w465:T1)
          }
          frame "Set Tunnel Speed Only" {
          }
          frame "Set Source Only" {
          }
          frame "Set Measurement Conditions" {
          }
          frame "Single Measurement" {
            n180 = Build Array("Averaging:Time:(mins)" ("Label for value"), "Filename:HD:Users" ("Label for value")) -> (w489:string[])
          }
          frame "Vertical Profile" {
            n181 = Build Array("Number:Of:Points" ("Label for value"), "Averaging:Time:(mins)" ("Label for value"), "Filename:HD:Users" ("Label for value")) -> (w496:string[])
          }
          frame "Lateral Profile" {
            n182 = Build Array("Number:Of:Points" ("Label for value"), "Averaging:Time:(mins)" ("Label for value"), "Filename:HD:Users" ("Label for value")) -> (w503:string[])
          }
          frame "Longitudinal Profile" {
            n183 = Build Array("Number:Of:Points" ("Label for value"), "Averaging:Time:(mins)" ("Label for value"), "Filename:HD:Users" ("Label for value")) -> (w510:string[])
          }
          frame "Explore Volume" {
            n184 = Unbundle By Name(w518) -> ("Specific Arguments"=w516:string)
            n185 = Build Array("Averaging:Time:(mins)" ("Label for value"), "Filename:HD:Users" ("Label for value")) -> (w523:string[])
            n186 = Fract/Exp String To Number(string=w516) -> (number=w515:dbl)  [unwired: 4 out]
            n187 = Greater Than 0?(x=w515) -> (x > 0?=w514:bool)
            n188 = Format Into String(format string="\"%s\" is an Incorrect Specific Argument. Please enter the radius of the volume in mm.\n", w516) -> (resulting string=w520:string)  [unwired: 2 in, 1 out]
            n189 = Select(t="", s=w514, f=w520) -> (s? t:f=w519:string)
          }
          frame "Multi-Axis Profile" {
            n190 = Unbundle By Name(w526) -> ("Spacing"=w529:T2)
            n191 = case shown="\"Gauss\"" w529 {
              tunnel: ["" "You are not allowed to specify gaussian spacing for a Multi-Axis profile.\n" "You are not allowed to specify Log spacing for a Multi-Axis profile.\n" "\"N/A\" is not a valid point spacing.\n"] -> w528
              frame "Linear", Default {
              }
              frame "Gauss" {
              }
              frame "Log" {
              }
              frame "N/A" {
              }
            }
            n192 = Build Array("Number:Of:Points" ("Label for value"), "Averaging:Time:(mins)" ("Label for value"), "Filename:HD:Users" ("Label for value")) -> (w531:string[])
          }
          frame "Traverse 3D Volume" {
            n193 = Build Array("Averaging:Time:(mins)" ("Label for value"), "Filename:HD:Users" ("Label for value")) -> (w541:string[])
          }
          frame "Auto Calibrate" {
            n194 = Unbundle By Name(w545) -> ("Filename"=w549:path, "Specific Arguments"=w580:string)
            n195 = call "Get_array_values_fr_String.vi"("String Value"=w580) -> ("Numeric Array"=w576:dbl[], "String array"=w563:string[])
            n196 = global read "Trav_pos_global.vi" "Work in Tunnel Coordinates?"() -> (w559:T7)
            n197 = Index Array(array=w563, index=0 ("Index")) -> (element=w562:string)
            n198 = Build Array("Tunnel Speed", "Traverse Position", "Concentration") -> (w561:string[])
            n199 = Build Array("Averaging:Time:(mins)" ("Label for value")) -> (w567:string[])
            n200 = Array Size(array=w576) -> (size(s)=w575:i32)
            n201 = call "Current_Filepath.vi"("Short_Name"="Cal" ("Data Type"), "Filename in"=w549, "Data Type"="Calibrations") -> ("Filename Out"=w547:path)  [unwired: 1 in, 1 out]
            n202 = Equal?(x=w559, y=Tunnel_Coordinates."Work in Model Coordinates" ("Work in Tunnel Coordinates?")) -> (x = y?=w553:bool)
            n203 = Search 1D Array(1D array=w561, element=w562) -> (index of element=w554:i32)  [unwired: 1 out]
            n204 = Equal?(x=2, y=w554) -> (x = y?=w556:bool)
            n205 = case shown="1" w554 {
              tunnel: [w610 w611] -> w566
              tunnel: w565 -> [w610 _]
              tunnel: w564 -> [_ w611]
              frame 0, Default {
              }
              frame 1 {
              }
            }
            n206 = Less?(x=w575, y=3) -> (x < y?=w571:bool)
            n207 = Equal To 0?(x=w554) -> (x = 0?=w572:bool)
            n208 = And(x=w553, y=w556) -> (x .and. y?=w555:bool)
            n209 = Greater Or Equal To 0?(x=w554) -> (x >= 0?=w552:bool)
            n210 = Compound Arithmetic op=AND(w571, w572) -> (w570:bool)
            n211 = case shown="True" w555 {
              tunnel: [w597 w602] -> w548
              tunnel: w545 -> [w597 w598]
              frame False {
              }
              frame True {
                n212 = global read "Extra_Commands_Global.vi" "Work in Tunnel Coordinates"() -> (w600:string)
                n213 = Unbundle By Name(w598) -> ("Extra Commands"=w599:string)
                n214 = call "Extra_Commands.vi"("String to Search"=w599, "Command"=w600) -> ("Command Found"=w601:bool)  [unwired: 1 in, 4 out]
                n215 = case shown="False" w601 {
                  tunnel: [w608 w609] -> w602
                  tunnel: w600 -> [w607 _]
                  tunnel: w599 -> [w606 _]
                  tunnel: w598 -> [w604 w609]
                  frame False {
                    n216 = Concatenate Strings(w607, "  " ("string"), w606) -> (w605:string)
                    n217 = Bundle By Name(cluster=w604, "Extra Commands"=w605) -> (w608:T1)
                  }
                  frame True {
                  }
                }
              }
            }
            n218 = Select(t="You need to enter the desired tunnel speeds in the \"Specfic Arguments\" Box   eg.  Tunnel Speed;1;2;3;4\n", s=w570, f="") -> (s? t:f=w568:string)
            n219 = call "Does_file_exist_(simple).vi"("Pathname"=w547) -> ("exists?"=w586:bool)
            n220 = case shown="False" w552 {
              tunnel: w561 -> [w588 _]
              tunnel: [w587 ""] -> w551
              frame False {
                n221 = for {
                  shift-right: [w593] -> w590
                  shift-left: "Incorrect Specific Argument. The options are: " -> [w594]
                  tunnel: w588 -> [w595] mode=indexing
                  w592 = "  " ("Substring")
                  n222 = Concatenate Strings(w594, w592, w595, w592) -> (w593:string)
                }
                n223 = Concatenate Strings(w590, "\r\n") -> (w587:string)
              }
              frame True {
              }
            }
            n224 = Select(t="", s=w586, f="The calibration file cannot be found.\n") -> (s? t:f=w582:string)
            n225 = Bundle By Name(cluster=w548, "Filename"=w547) -> (w546:T1)
            n226 = Concatenate Strings(w582, w568, w551) -> (w581:string)
          }
          frame "Meas Fast FID Bkgnd" {
            n227 = Unbundle By Name(w622) -> ("Specific Arguments"=w617:string)
            n228 = call "Get_array_values_fr_String.vi"("String Value"=w617) -> ("String array"=w616:string[])  [unwired: 1 out]
            n229 = Index Array(array=w616, index=0) -> (element=w614:string)
            n230 = Empty String/Path?(string/path=w614) -> (empty?=w620:bool)
            n231 = Build Array("Averaging:Time:(mins)" ("Label for value")) -> (w624:string[])
            n232 = Equal?(x=w614, y="Use Source Divertor Valve") -> (x = y?=w613:bool)
            n233 = Or(x=w620, y=w613) -> (x .or. y?=w619:bool)
            n234 = case shown="False" w619 {
              tunnel: ["Specific Argument should either be blank or\nUse Source Divertor Valve ; (wait time in seconds optional)" ""] -> w618
              frame False {
              }
              frame True {
              }
            }
          }
          frame "Check Beam Power" {
            n235 = Unbundle By Name(w629) -> ("Extra Commands"=w631:string, "Start X"=w636:dbl, "Start Y"=w634:dbl, "Start Z"=w635:dbl)
            n236 = global read "Extra_Commands_Global.vi" "Skip Traverse Position Demand"() -> (w632:string)
            n237 = call "Extra_Commands.vi"("String to Search"=w631, "Command"=w632) -> ("Command Found"=w630:bool)  [unwired: 1 in, 4 out]
            n238 = case shown="False" w630 {
              tunnel: w636 -> [w648 _]
              tunnel: w635 -> [w647 _]
              tunnel: w634 -> [w646 _]
              tunnel: "" -> [w643 w649]
              tunnel: [w642 w649] -> w628
              frame False {
                n239 = Build Array(w648, w646, w647) -> (w645:dbl[])
                n240 = Not A Number/Path/Refnum?(number/path/refnum=w645) -> (NaN/Path/Refnum?=w644:bool[])
                n241 = Or Array Elements(Boolean array=w644) -> (logical OR=w641:bool)
                n242 = Select(t="The start position is where the datum velocity measurement will be made. This should not contain NaNs.\n" ("f"), s=w641, f=w643) -> (s? t:f=w642:string)
              }
              frame True {
              }
            }
            n243 = Bundle By Name(cluster=w629, "Comments"="Start Position is the location of Datum Velocity Measurement") -> (w637:T1)
          }
          frame "Scanning Valve Measurement" {
            w663 = ext -0.5  # lo
            w664 = ext 47.5  # hi
            n244 = Unbundle By Name(w650) -> ("Specific Arguments"=w660:string)
            n245 = call "Get_array_values_fr_String.vi"("String Value"=w660) -> ("Numeric Array"=w659:dbl[], "String array"=w655:string[])
            n246 = Build Array("Averaging:Time:(mins)" ("Label for value"), "Filename:HD:Users" ("Label for value")) -> (w667:string[])
            n247 = Index Array(array=w655, index=0) -> (element=w654:string)
            n248 = Empty String/Path?(string/path=w654) -> (empty?=w652:bool)
            n249 = Index Array(array=w659, index=0) -> (element=w657:dbl)
            n250 = In Range and Coerce(upper limit=w664, x=w657, lower limit=w663) -> (In Range?=w653:bool)  [unwired: 1 out]
            n251 = Compound Arithmetic op=AND(invert w652, w653) -> (w651:bool)
            n252 = Select(t="", s=w651, f="Enter the scanning valve port number between 0 and 47 in the specific arguments box.\n") -> (s? t:f=w662:string)
          }
          frame "Set ADAM Ch" {
            n253 = Unbundle By Name(w687) -> ("Specific Arguments"=w694:string, "Extra Commands"=w682:string)
            n254 = while {
              shift-right: [w728] -> w693
              shift-left: _ -> [w721]
              shift-right: [w727] -> _
              shift-left: _ -> [w726]
              tunnel: w692 -> [w727]
              stop <- TRUE stop-if-true
              n255 = Array Size(array=w721) -> (size(s)=w725:i32)
              n256 = Less?(x=w727, y=w726) -> (x < y?=w723:bool)
              n257 = Equal To 0?(x=w725) -> (x = 0?=w724:bool)
              n258 = Or(x=w724, y=w723) -> (x .or. y?=w722:bool)
              n259 = case shown="True" w722 {
                tunnel: [w729 w730] -> w728
                tunnel: w721 -> [w729 _]
                frame False {
                }
                frame True {
                  n260 = call "Get_ADAM_Ch_names_client.vi"("Channel names set"=Channel_names."Active + Off") -> ("Ch names"=w730:string[])
                }
              }
            }
            n261 = call "Get_array_values_fr_String.vi"("String Value"=w682) -> ("Numeric Array"=w678:dbl[])  [unwired: 1 out]
            n262 = call "Get_array_values_fr_String.vi"("String Value"=w694) -> ("String array"=w679:string[])  [unwired: 1 out]
            n263 = for {
              tunnel: w693 -> [w702]
              tunnel: w679 -> [w701] mode=indexing
              tunnel: w678 -> [w697]
              tunnel: [w699] -> w681 mode=indexing
              tunnel: [w698] -> w680 mode=indexing
              i -> [w696]
              n264 = Index Array(array=w697, index=w696) -> (element=w700:dbl)
              n265 = Search 1D Array(1D array=w702, element=w701) -> (index of element=w703:i32)  [unwired: 1 out]
              n266 = Not A Number/Path/Refnum?(number/path/refnum=w700) -> (NaN/Path/Refnum?=w698:bool)
              n267 = Greater Or Equal To 0?(x=w703) -> (x >= 0?=w699:bool)
            }
            n268 = Array Size(array=w679) -> (size(s)=w673:i32)
            n269 = Array Size(array=w678) -> (size(s)=w677:i32)
            n270 = Not Equal?(x=w673, y=w677) -> (x != y?=w675:bool)
            n271 = Greater Than 0?(x=w673) -> (x > 0?=w671:bool)
            n272 = Or Array Elements(Boolean array=w680) -> (logical OR=w676:bool)
            n273 = And Array Elements(Boolean array=w681) -> (logical AND=w672:bool)
            n274 = Or(x=w675, y=w676) -> (x .or. y?=w674:bool)
            n275 = Select(t="You have not specified a Value to Set the ADAM channel to.\nPlease give the values separated by ; in the Extra Commands string", s=w674, f="") -> (s? t:f=w683:string)
            n276 = And(x=w671, y=w672) -> (x .and. y?=w670:bool)
            n277 = case shown="True" w670 {
              tunnel: w693 -> [w714 _]
              tunnel: w679 -> [w706 w716]
              tunnel: w692 -> [w712 _]
              tunnel: [w710 FALSE ("Cancel")] -> w691
              tunnel: w687 -> [w708 w718]
              tunnel: [w707 w717] -> w686
              frame False {
                n278 = Format Into String(format string="Please Select the ADAM Channels that you want to set in row %d", w712) -> (resulting string=w711:string)  [unwired: 2 in, 1 out]
                n279 = call "Select_Strings.vi"("Available Ch names"=w714, "Message"=w711, "Selector mode"=T8."One or more", "Desired Ch names (in)"=w706) -> ("Cancel"=w710:bool, "Selected Channel Names"=w705:string[])  [unwired: 3 out]
                n280 = call "Put_Array_into_String.vi"("String array"=w705) -> ("String Value"=w704:string)
                n281 = Bundle By Name(cluster=w708, "Specific Arguments"=w704) -> (w707:T1)
              }
              frame True {
                n282 = call "Put_Array_into_String.vi"("String array"=w716) -> ("String Value"=w715:string)
                n283 = Bundle By Name(cluster=w718, "Specific Arguments"=w715) -> (w717:T1)
              }
            }
            n284 = Select(t="Close Front Panel", s=w691, f=w689) -> (s? t:f=w690:string)
          }
          frame "Run VI Named:" {
            w743 = "Run_VI_Named_specific.vi"
            n285 = Unbundle By Name(w738) -> ("Specific Arguments"=w746:string)
            n286 = global read "Constants_global.vi" "Run VI Folder"() -> (w744:path)
            n287 = Match Pattern(string=w746, regular expression=";") -> (before substring=w747:string)  [unwired: 4 out]
            n288 = call <vilib>:"Trim Whitespace.vi"("string"=w747) -> ("trimmed string"=w739:string)  [unwired: 1 in]
            n289 = call "Run_VI_Named_specific.vi"("Run VI Named String"=w739, "Multi Run Row"=w738) -> ("Checks"=w733:string[], "Error String"=w732:string, "Check for start NaNs?"=w737:bool)  [unwired: 7 out]
            n290 = Select(t="Check for Start NaNs" ("Label for value"), s=w737, f=w735) -> (s? t:f=w734:string)
            n291 = Build Path(base path=w744, name or relative path=w739) -> (appended path=w750:path)
            n292 = Not Equal?(x=w739, y=w743) -> (x != y?=w742:bool)
            n293 = call "Does_file_exist_(simple).vi"("Pathname"=w750) -> ("exists?"=w741:bool)
            n294 = And(x=w741, y=w742) -> (x .and. y?=w740:bool)
            n295 = case shown="False" w740 {
              tunnel: [w757 ""] -> w745
              tunnel: w744 -> [w753 _]
              tunnel: w743 -> [w751 _]
              frame False {
                w755 = "\r\n"
                n296 = Build Array(w751) -> (w752:string[])
                n297 = call "List_files_in_order_of_age.vi"("Files to Hide"=w752, "Folder"=w753) -> ("file names"=w754:string[])
                n298 = for {
                  shift-right: [w761] -> w758
                  shift-left: "Cannot find the VI to run. Specific Argument options are:" -> [w762]
                  tunnel: w754 -> [w763] mode=indexing
                  w760 = "  " ("Substring")
                  n299 = Concatenate Strings(w762, w760, w763, w760) -> (w761:string)
                }
                n300 = Concatenate Strings(w758, w755, "Please place one of these strings in the \"Specific Argument\" field.", w755) -> (w757:string)
              }
              frame True {
              }
            }
            n301 = Concatenate Strings(w732, w745) -> (w749:string)
          }
          frame "Wait (minutes)" {
            n302 = Unbundle By Name(w766) -> ("Specific Arguments"=w767:string)
            n303 = call "Wait_Case_Arg.vi"("Specific Argument"=w767) -> ("Error Comments"=w768:string)  [unwired: 1 in, 4 out]
          }
          frame "Send Message" {
          }
          frame "Synchronize With:" {
            n304 = local read "Current Sync Number"() -> (w776:i32)
            n305 = call "Synchronize_Prog_Arg.vi"("Execution Row"=w775) -> ("Error Comments"=w778:string, "Sync No"=w784:i32)  [unwired: 3 out]
            n306 = Equal?(x=w784, y=w776) -> (x = y?=w783:bool)
            n307 = Format Into String(format string="This should be Synchroisation number %d.\n" ("Format String"), w776) -> (resulting string=w781:string)  [unwired: 2 in, 1 out]
            n308 = Select(t="", s=w783, f=w781) -> (s? t:f=w779:string)
            n309 = Concatenate Strings(w779, w778) -> (w777:string)
          }
          frame "Fall Back to this Row" {
          }
          frame "Turn Off Row Repeating" {
          }
          frame "Blank Row" {
            n310 = Unbundle By Name(w797) -> ("Comments"=w803:string)
            n311 = Match Pattern(string=w803, regular expression="(No Match Info)") -> (before substring=w796:string, after substring=w800:string)  [unwired: 3 out]
            n312 = Empty String/Path?(string/path=w800) -> (empty?=w801:bool)
            n313 = Bundle By Name(cluster=w797, "Comments"=w796) -> (w795:T1)
            n314 = Select(t=w800, s=w801, f="The Row Type Selector \"%s\" was not matched. Please select the desired type.\n") -> (s? t:f=w799:string)
          }
        }
        "Checks" <- w454
        n315 = Concatenate Strings(w457, w458) -> (w456:string)
      }
      frame "Sort out start and end positions" {
        n316 = Unbundle By Name(w811) -> ("Start X"=w823:dbl, "Start Y"=w822:dbl, "Start Z"=w821:dbl, "End X"=w820:dbl, "End Y"=w819:dbl, "End Z"=w818:dbl, "Extra Commands"=w807:string)
        n317 = call "Which_Trav_Setup.vi"("Extra Command String"=w807) -> ("Traverse Setups"=w805:string[])
        n318 = Build Array(w823, w822, w821) -> (w814:dbl[])
        n319 = Build Array(w820, w819, w818) -> (w813:dbl[])
        n320 = Index Array(array=w805) -> (element=w806:string)  [unwired: 1 in]
        n321 = call "Rig_Pict_Display_Pref.vi"("Traverse Name"=w806) -> ("Which Axis is vertical?"=w817:enum16{"X Axis", "Y Axis", "Z Axis"})  [unwired: 7 out]
        n322 = case shown="\"Longitudinal Profile\"" w812 {
          tunnel: [w863 FALSE w879 w892 FALSE] -> w826
          tunnel: [w862 FALSE w878 w891 FALSE] -> w825
          tunnel: [w861 FALSE w877 w890 FALSE] -> w824
          tunnel: w817 -> [w860 _ w876 w889 _]
          frame "Vertical Profile" {
            n323 = case shown="\"Z Axis\"" w860 {
              tunnel: [FALSE TRUE TRUE] -> w863
              tunnel: [TRUE FALSE TRUE] -> w862
              tunnel: [TRUE TRUE FALSE] -> w861
              frame "X Axis" {
              }
              frame "Y Axis" {
              }
              frame "Z Axis" {
              }
            }
          }
          frame "Auto Calibrate" {
          }
          frame "Lateral Profile" {
            n324 = case shown="\"Y Axis\"" w876 {
              tunnel: [TRUE TRUE TRUE] -> w879
              tunnel: [TRUE TRUE FALSE] -> w878
              tunnel: [FALSE FALSE TRUE] -> w877
              frame "X Axis" {
              }
              frame "Y Axis" {
              }
              frame "Z Axis" {
              }
            }
          }
          frame "Longitudinal Profile" {
            n325 = case shown="\"Y Axis\"" w889 {
              tunnel: [FALSE FALSE FALSE] -> w892
              tunnel: [TRUE TRUE TRUE] -> w891
              tunnel: [TRUE TRUE TRUE] -> w890
              frame "X Axis" {
              }
              frame "Y Axis" {
              }
              frame "Z Axis" {
              }
            }
          }
          frame "Multi-Axis Profile", Default {
          }
        }
        n326 = Build Array(w826, w825, w824) -> (w815:bool[])
        "Fixed Axis" <- w815
        n327 = for {
          tunnel: w815 -> [w833] mode=indexing
          tunnel: w814 -> [w832] mode=indexing
          tunnel: w813 -> [w831] mode=indexing
          shift-right: [w828] -> w810
          shift-left: w811 -> [w829]
          i -> [w830]
          n328 = case shown="True" w833 {
            tunnel: w832 -> [_ w839]
            tunnel: w831 -> [_ w838]
            tunnel: w830 -> [_ w837]
            tunnel: w829 -> [w834 w836]
            tunnel: [w834 w835] -> w828
            frame False {
            }
            frame True {
              n329 = Not A Number/Path/Refnum?(number/path/refnum=w839) -> (NaN/Path/Refnum?=w840:bool)
              n330 = Not A Number/Path/Refnum?(number/path/refnum=w838) -> (NaN/Path/Refnum?=w842:bool)
              n331 = Exclusive Or(1:w842, 2:w840) -> (0:w841:bool)
              n332 = case shown="True" w841 {
                tunnel: w840 -> [_ w850]
                tunnel: w839 -> [_ w849]
                tunnel: w838 -> [_ w848]
                tunnel: w837 -> [_ w847]
                tunnel: w836 -> [w843 w846]
                tunnel: [w843 w845] -> w835
                frame False {
                }
                frame True {
                  n333 = Select(t=w848, s=w850, f=w849) -> (s? t:f=w844:dbl)
                  n334 = case shown="2" w847 {
                    tunnel: w846 -> [w853 w856 w859]
                    tunnel: [w852 w855 w858] -> w845
                    tunnel: w844 -> [w851 w854 w857]
                    frame 0, Default {
                      n335 = Bundle By Name(cluster=w853, "Start X"=w851, "End X"=w851) -> (w852:T1)
                    }
                    frame 1 {
                      n336 = Bundle By Name(cluster=w856, "Start Y"=w854, "End Y"=w854) -> (w855:T1)
                    }
                    frame 2 {
                      n337 = Bundle By Name(cluster=w859, "Start Z"=w857, "End Z"=w857) -> (w858:T1)
                    }
                  }
                }
              }
            }
          }
        }
      }
      frame "Check for position NaNs" {
        n338 = global read "Extra_Commands_Global.vi" "Skip Traverse Position Demand"() -> (w908:string)
        n339 = Unbundle By Name(w911) -> ("Extra Commands"=w907:string, "Start X"=w920:dbl, "Start Y"=w918:dbl, "Start Z"=w919:dbl, "End X"=w917:dbl, "End Y"=w916:dbl, "End Z"=w915:dbl)
        n340 = call "Extra_Commands.vi"("String to Search"=w907, "Command"=w908) -> ("Command Found"=w905:bool)  [unwired: 1 in, 4 out]
        n341 = case shown="False" w905 {
          tunnel: w920 -> [w935 _]
          tunnel: w919 -> [w934 _]
          tunnel: w918 -> [w933 _]
          tunnel: w917 -> [w932 _]
          tunnel: w916 -> [w931 _]
          tunnel: w915 -> [w930 _]
          tunnel: [w926 w936] -> w914
          tunnel: [w925 TRUE] -> w913
          tunnel: "" -> [w924 w936]
          frame False {
            n342 = Build Array(w935, w933, w934, w932, w931, w930) -> (w929:dbl[])
            n343 = Not A Number/Path/Refnum?(number/path/refnum=w929) -> (NaN/Path/Refnum?=w928:bool[])
            n344 = Or Array Elements(Boolean array=w928) -> (logical OR=w925:bool)
            n345 = Select(t="Some of the Start and End positions are NaN.\n" ("f"), s=w925, f=w924) -> (s? t:f=w926:string)
          }
          frame True {
          }
        }
        n346 = case shown="\"Set Tunnel Speed Only\", Default" w909 {
          tunnel: w913 -> [_ w942]
          tunnel: ["Check source details" ("t") w941] -> w912
          frame "Multi-Axis Profile" {
          }
          frame "Set Tunnel Speed Only", Default {
            n347 = Select(t="Check source details", s=w942, f="Check profile rows") -> (s? t:f=w941:string)
          }
        }
        n348 = Concatenate Strings(w922, w914) -> (w921:string)
      }
      frame "Check for Start NaNs" {
        n349 = Unbundle By Name(w948) -> ("Extra Commands"=w944:string, "Start X"=w953:dbl, "Start Y"=w951:dbl, "Start Z"=w952:dbl)
        n350 = global read "Extra_Commands_Global.vi" "Skip Traverse Position Demand"() -> (w945:string)
        n351 = call "Extra_Commands.vi"("String to Search"=w944, "Command"=w945) -> ("Command Found"=w943:bool)  [unwired: 1 in, 4 out]
        n352 = case shown="True" w943 {
          tunnel: w953 -> [w965 _]
          tunnel: w952 -> [w964 _]
          tunnel: w951 -> [w963 _]
          tunnel: "" -> [w960 w966]
          tunnel: [w958 w966] -> w949
          frame False {
            n353 = Build Array(w965, w963, w964) -> (w962:dbl[])
            n354 = Not A Number/Path/Refnum?(number/path/refnum=w962) -> (NaN/Path/Refnum?=w961:bool[])
            n355 = Or Array Elements(Boolean array=w961) -> (logical OR=w957:bool)
            n356 = Select(t="Some of the Start coordinates are NaN.\n" ("f"), s=w957, f=w960) -> (s? t:f=w958:string)
          }
          frame True {
          }
        }
        n357 = Concatenate Strings(w955, w949) -> (w954:string)
      }
      frame "Check profile rows" {
        n358 = call "Create_Pos_array.vi"("Traverse line"=w976) -> ("Traverse line Out"=w975:T1, "Error Messages"=w974:string)  [unwired: 7 out]
        n359 = Unbundle By Name(w976) -> ("Start X"=w998:dbl, "Start Y"=w997:dbl, "Start Z"=w996:dbl, "End X"=w995:dbl, "End Y"=w994:dbl, "End Z"=w993:dbl, "Specific Arguments"=w987:string, "Spacing"=w982:T2, "No. of pts."=w981:i32)
        n360 = local read "Fixed Axis"() -> (w980:bool[])
        n361 = Build Array(w998, w997, w996) -> (w978:dbl[])
        n362 = Build Array(w995, w994, w993) -> (w979:dbl[])
        n363 = case shown="\"Linear\"" w982 {
          tunnel: w987 -> [_ _ _ _ w1033]
          tunnel: ["" w1006 "\"N/A\" is not a valid point spacing.\n" "" w1028] -> w986
          tunnel: w981 -> [_ _ _ _ w1032]
          tunnel: w980 -> [_ w1004 _ _ _]
          tunnel: w979 -> [_ w1011 _ _ _]
          tunnel: w978 -> [_ w1010 _ _ _]
          frame "Linear" {
          }
          frame "Log" {
            n364 = for {
              tunnel: w1011 -> [w1015] mode=indexing
              tunnel: w1010 -> [w1014] mode=indexing
              tunnel: [w1013] -> w1009 mode=indexing
              tunnel: w1004 -> [w1012] mode=indexing
              n365 = case shown="False" w1012 {
                tunnel: w1015 -> [w1021 _]
                tunnel: w1014 -> [w1020 _]
                tunnel: [w1016 FALSE] -> w1013
                frame False {
                  w1019 = 0.001 ("y")
                  n366 = Less?(x=w1021, y=w1019) -> (x < y?=w1017:bool)
                  n367 = Less?(x=w1020, y=w1019) -> (x < y?=w1018:bool)
                  n368 = Or(x=w1017, y=w1018) -> (x .or. y?=w1016:bool)
                }
                frame True {
                }
              }
            }
            n369 = Or Array Elements(Boolean array=w1009) -> (logical OR=w1008:bool)
            n370 = Select(t="For log spacing, Start & End positions must be greater than 0.0001.", s=w1008, f="") -> (s? t:f=w1006:string)
          }
          frame "N/A" {
          }
          frame "Gauss" {
          }
          frame "Specified" {
            n371 = call "Get_array_values_fr_String.vi"("String Value"=w1033) -> ("Numeric Array"=w1027:dbl[])  [unwired: 1 out]
            n372 = Array Size(array=w1027) -> (size(s)=w1026:i32)
            n373 = Decrement(x=w1026) -> (x-1=w1025:i32)
            n374 = Equal?(x=w1025, y=w1032) -> (x = y?=w1031:bool)
            n375 = Select(t="", s=w1031, f="The No of points and No of Arguments do not match.\n") -> (s? t:f=w1028:string)
          }
        }
        n376 = for {
          tunnel: w980 -> [w1039] mode=indexing
          tunnel: w978 -> [w1038] mode=indexing
          tunnel: w979 -> [w1037] mode=indexing
          tunnel: [w1036] -> w992 mode=indexing
          shift-right: [w1034] -> w971
          shift-left: bool[] [] -> [w1035]
          n377 = case shown="False" w1039 {
            tunnel: w1038 -> [w1043 w1049]
            tunnel: w1037 -> [w1044 w1048]
            tunnel: [TRUE w1047] -> w1036
            tunnel: w1035 -> [w1041 w1046]
            tunnel: [w1040 w1046] -> w1034
            frame False {
              n378 = Not Equal?(x=w1043, y=w1044) -> (x != y?=w1042:bool)
              n379 = Build Array (concatenate)(w1041, w1042) -> (w1040:bool[])
            }
            frame True {
              n380 = Equal?(x=w1049, y=w1048) -> (x = y?=w1047:bool)
            }
          }
        }
        n381 = Array Size(array=w971) -> (size(s)=w970:i32)
        n382 = And Array Elements(Boolean array=w992) -> (logical AND=w991:bool)
        n383 = Or Array Elements(Boolean array=w971) -> (logical OR=w968:bool)
        n384 = Not Equal To 0?(x=w970) -> (x != 0?=w969:bool)
        n385 = And(x=w968, y=w969) -> (x .and. y?=w967:bool)
        n386 = Select(t="", s=w991, f="This profile moves more than one axis.\n") -> (s? t:f=w988:string)
        n387 = Select(t="", s=w967, f="The start and end points are the same for this profile.\n") -> (s? t:f=w984:string)
        n388 = Concatenate Strings(w974, w984, w988, w986) -> (w1001:string)
        n389 = Concatenate Strings(w1000, w1001) -> (w999:string)
      }
      frame "Check source details" {
        n390 = Unbundle By Name(w1061) -> ("Emission Rate (l/min)"=w1063:dbl, "Density Ratio"=w1053:string)  [unwired: 1 out]
        n391 = Empty String/Path?(string/path=w1053) -> (empty?=w1054:bool)
        n392 = Equal?(x=w1053, y="---------" ("f")) -> (x = y?=w1052:bool)
        n393 = Or(x=w1054, y=w1052) -> (x .or. y?=w1051:bool)
        n394 = Greater Than 0?(x=w1063) -> (x > 0?=w1058:bool)
        n395 = And(x=w1058, y=w1051) -> (x .and. y?=w1062:bool)
        n396 = case shown="False" w1062 {
          tunnel: w1061 -> [w1066 w1069]
          tunnel: [w1066 w1067] -> w1060
          frame False {
          }
          frame True {
            (unwired) "The Density Ratio Box should contain either:\nCarrier 1 Only\nCarrier 2 Only\nor the relative density ratio of the mixed gas with respect to air" ("f")
            n397 = Bundle By Name(cluster=w1069, "Density Ratio"="Carrier 1 Only") -> (w1067:T1)
          }
        }
        n398 = Select(t="Check source detail 2", s=w1058, f="check entered filename etc") -> (s? t:f=w1056:string)
      }
      frame "Check source detail 2" {
        n399 = Unbundle By Name(w1093) -> ("Trace Gas Concentration (%)"=w1094:dbl, "Density Ratio"=w1095:string)
        n400 = To Upper Case(1:w1095) -> (0:w1078:string)
        n401 = To Upper Case(1:"Carrier 1 Only") -> (0:w1080:string)
        n402 = To Upper Case(1:"Carrier 2 Only") -> (0:w1079:string)
        n403 = In Range and Coerce(upper limit=ext 3.01 ("hi"), x=w1094, lower limit=ext 0.0 ("lo")) -> (In Range?=w1075:bool)  [unwired: 1 out]
        n404 = Equal?(x=w1078, y=w1080) -> (x = y?=w1085:bool)
        n405 = Equal?(x=w1078, y=w1079) -> (x = y?=w1084:bool)
        n406 = Fract/Exp String To Number(string=w1078) -> (number=w1086:dbl)  [unwired: 4 out]
        n407 = In Range and Coerce(upper limit=ext 10.0 ("hi"), x=w1086, lower limit=ext 0.05 ("lo")) -> (In Range?=w1083:bool)  [unwired: 1 out]
        n408 = Compound Arithmetic op=OR(w1085, w1084, w1083) -> (w1070:bool)
        n409 = Select(t="", s=w1075, f="The Trace Gas Concentration must be within the range of 0 to 3%.\n") -> (s? t:f=w1071:string)
        n410 = Select(t="", s=w1070, f="The Density Ratio Box should contain either:\nCarrier 1 Only\nCarrier 2 Only\nor the relative density ratio of the mixed gas with respect to air") -> (s? t:f=w1072:string)
        n411 = Concatenate Strings(w1071, w1072) -> (w1096:string)
        n412 = Concatenate Strings(w1098, w1096) -> (w1097:string)
      }
      frame "check entered filename etc" {
        n413 = local read "Checks"() -> (w1111:string[])
        n414 = for {
          tunnel: w1111 -> [w1118] mode=indexing
          tunnel: [w1123] -> w1112 mode=indexing
          tunnel: w1108 -> [w1122]
          shift-right: [w1120] -> w1102
          shift-left: w1103 -> [w1121]
          tunnel: [w1119] -> w1101 mode=indexing
          n415 = case shown="\"Filename:HD:Users\"" w1118 {
            tunnel: w1121 -> [w1125 w1133 w1156 w1171]
            tunnel: [w1126 w1136 w1162 w1167] -> w1123
            tunnel: w1122 -> [_ _ w1165 _]
            tunnel: [w1125 w1133 w1154 w1171] -> w1120
            tunnel: [TRUE ("cancelled") TRUE ("cancelled") w1149 TRUE ("cancelled")] -> w1119
            tunnel: w1118 -> [_ _ _ w1169]
            frame "Number:Of:Points" {
              n416 = Unbundle By Name(w1125) -> ("No. of pts."=w1128:i32)
              n417 = Greater?(x=w1128, y=0) -> (0:w1130:bool)
              n418 = Select(t="", s=w1130, f="For a profile the number of points should be more than 0.\n" ("Format String")) -> (s? t:f=w1126:string)
            }
            frame "Averaging:Time:(mins)" {
              n419 = Unbundle By Name(w1133) -> ("Averaging time (min)"=w1135:dbl)
              n420 = Greater Than 0?(x=w1135) -> (x > 0?=w1134:bool)
              n421 = Select(t="", s=w1134, f="The averaging time should be greater than zero.\n" ("Format String")) -> (s? t:f=w1136:string)
            }
            frame "Filename:HD:Users" {
              w1163 = FALSE  # Show Error handler
              n422 = Unbundle By Name(w1156) -> ("Filename"=w1140:path, "Row No"=w1151:i32, "Row Type Selector"=w1147:T3)
              n423 = call "Row_type_selector_string.vi"("Mode"=w1147) -> ("Output string"=w1146:string)
              n424 = call "Current_Filepath.vi"("Short_Name"="Res" ("Data Type"), "Filename in"=w1140, "Data Type"="Results") -> ("Filename Out"=w1141:path)  [unwired: 1 in, 1 out]
              n425 = Path To String(path=w1141) -> (string=w1160:string)
              n426 = Not A Number/Path/Refnum?(number/path/refnum=w1141) -> (NaN/Path/Refnum?=w1144:bool)
              n427 = Equal?(x=Multi_run_mode."Run VI Named:" ("Mode"), y=w1165) -> (x = y?=w1164:bool)
              n428 = Match Pattern(string=w1160, regular expression="-------" ("f")) -> (match substring=w1159:string)  [unwired: 4 out]
              n429 = Empty String/Path?(string/path=w1159) -> (empty?=w1145:bool)
              n430 = Format Into String(format string=" For Row  %d %s." ("Comment"), w1151, w1146) -> (resulting string=w1150:string)  [unwired: 2 in, 1 out]
              n431 = Compound Arithmetic op=AND(w1145, invert w1144) -> (w1143:bool)
              n432 = Select(t=w1141, s=w1143, f=path "") -> (s? t:f=w1158:path)
              n433 = call "Results_filename_checker.vi"("Filelength"=45, "Warn if Already Exists"=w1164, "Comment"=w1150, "Show Error handler"=w1163, "Results file"=w1158) -> ("Error String"=w1162:string, "cancelled"=w1153:bool, "Results file output"=w1155:path)  [unwired: 1 out]
              n434 = Bundle By Name(cluster=w1156, "Filename"=w1155) -> (w1154:T1)
              n435 = Not(x=w1153) -> (.not. x?=w1149:bool)
            }
            frame "No Match", Default {
              n436 = Concatenate Strings(w1169, " Has not been programmed.\n" ("string")) -> (w1167:string)
            }
          }
        }
        n437 = local read "Editted Row"() -> (w1105:bool)
        n438 = And Array Elements(Boolean array=w1101) -> (logical AND=w1100:bool)
        n439 = Concatenate Strings(w1112) -> (w1110:string)
        n440 = Concatenate Strings(w1109, w1110) -> (w1104:string)
        n441 = Empty String/Path?(string/path=w1104) -> (empty?=w1107:bool)
        n442 = case shown="False" w1107 {
          tunnel: ["Open Front Panel" w1116] -> w1106
          tunnel: w1105 -> [_ w1117]
          frame False {
          }
          frame True {
            n443 = Select(t="Close Front Panel", s=w1117, f="End") -> (s? t:f=w1116:string)
          }
        }
      }
      frame "Open Front Panel" {
        w1176 = TRUE  # Front Panel Window:Open
        n444 = Current VI's Path() -> (path=w1177:path)
        n445 = call "Open_Close_Front_Panel.ph.vi"("Front Panel Window:Open"=w1176, "VI path"=w1177) -> ()  [unwired: 2 out]
        n446 = local write "Editted Row"(TRUE ("Editted Row")) -> ()
        n447 = local write "Execution Row"(w1173) -> ()
      }
      frame "What to do next?" {
        w1187 = ""
        w1185 = "[\r\n]"
        n448 = local read "Execution Row"() -> (w1183:T1)
        n449 = Unbundle By Name(w1183) -> ("Row Type Selector"=w1199:T3, "Specific Arguments"=w1194:string, "Extra Commands"=w1192:string, "Density Ratio"=w1186:string)
        n450 = Wait Until Next ms Multiple(millisecond multiple=u32 100) -> ()  [unwired: 1 out]
        n451 = Not Equal?(x=Multi_run_mode."Blank Row" ("Mode"), y=w1199) -> (x != y?=w1195:bool)
        n452 = call "Replace_Character.vi"("Replace with"=w1187, "Input String"=w1194, "Search For"=w1185) -> ("Output string"=w1193:string)  [unwired: 1 out]
        n453 = call "Replace_Character.vi"("Replace with"=w1187, "Input String"=w1192, "Search For"=w1185) -> ("Output string"=w1191:string)  [unwired: 1 out]
        n454 = call "Replace_Character.vi"("Replace with"=w1187, "Input String"=w1186, "Search For"=w1185) -> ("Output string"=w1184:string)  [unwired: 1 out]
        n455 = Compound Arithmetic op=OR("Edit in Excel", "OK") -> (w1196:bool)
        n456 = Bundle By Name(cluster=w1183, "Specific Arguments"=w1193, "Extra Commands"=w1191, "Density Ratio"=w1184) -> (w1181:T1)
        n457 = Compound Arithmetic op=AND(w1196, w1195) -> (w1189:bool)
        n458 = Not Equal?(x=w1181, y=w1183) -> (x != y?=w1182:bool)
        n459 = Not(x="Edit in Excel") -> (.not. x?=w1180:bool)
        n460 = case shown="True" w1182 {
          tunnel: w1181 -> [_ w1203]
          frame False {
          }
          frame True {
            n461 = local write "Execution Row"(w1203) -> ()
          }
        }
        n462 = case shown="True" w1180 {
          tunnel: ["Close Front Panel" w1208] -> w1188
          tunnel: w1189 -> [_ w1207]
          frame False {
          }
          frame True {
            n463 = Select(t="Clean Up Row", s=w1207, f="What to do next?") -> (s? t:f=w1208:string)
          }
        }
        "Error Comments" <- w1190
      }
      frame "Clean Up Row" {
        n464 = call "Traverse_Control_Ch_Names.vi"("Mode"=T4."All Channel Names") -> ("Channel names"=w1217:string[])  [unwired: 1 in]
        n465 = call "Trav_Cluster_to_Row.vi"("Traverse line in"=w1212, "Row Number"=w1213, "Channel names"=w1217) -> ("Traverse line Out"=w1215:T1)  [unwired: 4 out]
      }
      frame "Close Front Panel" {
        w1221 = FALSE  # Front Panel Window:Open
        n466 = Current VI's Path() -> (path=w1222:path)
        n467 = call "Open_Close_Front_Panel.ph.vi"("Front Panel Window:Open"=w1221, "VI path"=w1222) -> ()  [unwired: 2 out]
      }
      frame "End" {
        n468 = local read "Editted Row"() -> (w1230:bool)
        n469 = case shown="True" w1230 {
          tunnel: w1229 -> [w1233 w1236]
          tunnel: [w1233 w1235] -> w1227
          tunnel: w1228 -> [_ w1234]
          frame False {
          }
          frame True {
            n470 = call "Traverse_Control_Ch_Names.vi"("Mode"=T4."All Channel Names") -> ("Channel names"=w1237:string[])  [unwired: 1 in]
            n471 = call "Trav_Cluster_to_Row.vi"("Traverse line in"=w1236, "Row Number"=w1234, "Channel names"=w1237) -> ("Traverse line Out"=w1235:T1)  [unwired: 4 out]
          }
        }
        n472 = local write "Error Comments"(w1231) -> ()
      }
    }
    "Traverse line Out" <- w8
  }
  "Execution Row Out" <- w2
  "Continue?" <- w1
